vi "Sleep.vi"(8 "error in (no error)":errorcluster, 11 "CIFCorePlugin in":refnum<class "CIFCorePlugin.lvclass">) -> (0 "error out":errorcluster, 2 "Housekeep only":bool, 3 "CIFCorePlugin out":refnum<class "CIFCorePlugin.lvclass">)   [LabVIEW 2021, in "CIFCorePlugin.lvclass"]
uses:
  CIFCorePlugin.lvclass
  CIFCorePlugin.lvclass/CIFCorePlugin.ctl
  CIFUtilities/CIFClocks/Typedef/Errors.ctl
  Accessors/Read Sleep Limits (ns).vi
  Accessors/Timestamps/Write Target Wake TS.vi
  Accessors/Get Time.vi
  Accessors/Timestamps/Read Running TS.vi
  Accessors/Read Running Internal Data.vi
  Accessors/Read Timing Override.vi
  Accessors/Read Common Config.vi
  CIFUtilities/CIFClocks/Core/Get Time.vi
  Common/Utilities/Append Error Location.vi
  CIFUtilities/CIFClocks/Time Conversion/LabVIEW Time to UTC Time.vi
  Common/CIFCoreCommon.lvlib
  CIFUtilities/CIFClocks/CIFClocks.lvlib
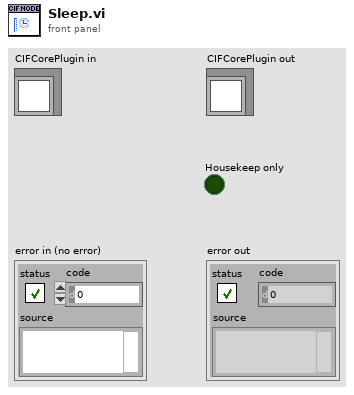
[diagram p1: front panel]
types:
  T1 = typedef "CIFCoreCommon.lvlib/Errors.ctl" = enum16{"Invalid Clock ID", "Long Sleep", "gRPC Server Not Found", "Config Parse", "Timestamp Wrap", "Delayed Execution", "Duplicate Channel", "Missing Channel", "Incorrect Type", "Unregistered Enum"}
  T2 = typedef "CIFCoreCommon.lvlib/Timing Overrides.ctl" = cluster{"Override Timing":bool, "Skip Sleep":bool, "Period (s)":dbl}
  T3 = typedef "CIFCorePlugin.lvclass/Running Internal Data.ctl" = cluster{"Refresh":bool, "Iterations":i64, "Housekeep only":bool, "Configured period (ns)":i64}
  T4 = typedef "CIFCoreCommon.lvlib/Common Plugin Configuration.ctl" = cluster{"Period (s)":dbl, "Offset (us)":i32, "ClockID":u8, "Priority":i32, "Processor":i32}
  T5 = typedef "CIFClocks.lvlib/Future Time Event Limits.ctl" = cluster{"Maximum":u64, "Minimum":u64}
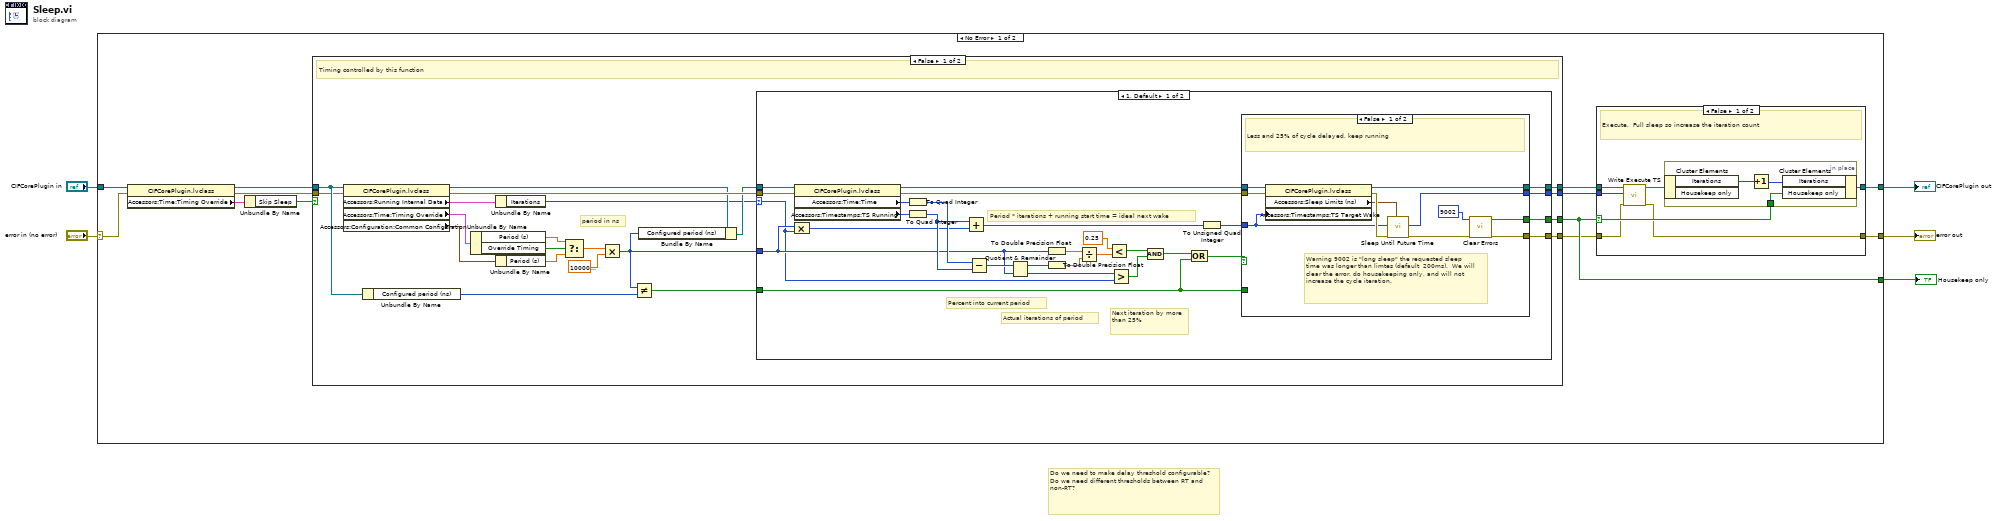
[diagram p0: block diagram]
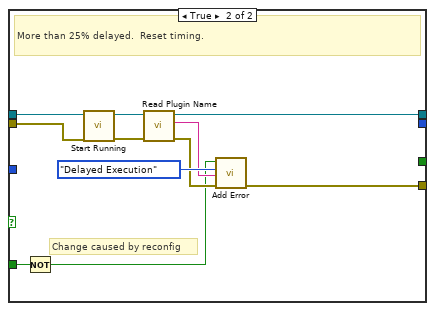
[diagram p2: hidden frame]
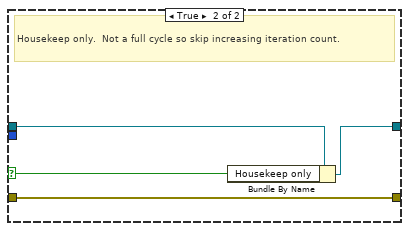
[diagram p5: hidden frame]
diagram:
  # "Do we need to make delay threshold configurable?  Do we need different thresholds between RT and non-RT?"
  n1 = case shown="No Error" "error in (no error)" {
    selector: "error in (no error)" -> [w10 w109]
    tunnel: [w12 w109] -> w4
    tunnel: [w16 w108] -> w2
    tunnel: "CIFCorePlugin in" -> [w11 w108]
    tunnel: [w15 _] -> w1
    frame No Error {
      n2 = property class="CIFCorePlugin.lvclass"(reference=w11, error in=w10) -> (reference out=w9:refnum<class "CIFCorePlugin.lvclass">, error out=w8:errorcluster, "Accessors:Time:Timing Override"=w7:T2)
      n3 = Unbundle By Name(w7) -> ("Skip Sleep"=w6:bool)
      n4 = case shown="False" w6 {
        tunnel: [w38 w93] -> w17
        tunnel: [w24 _] -> w15
        tunnel: [w21 _] -> w14
        tunnel: [w20 w92] -> w13
        tunnel: w9 -> [w19 w93]
        tunnel: w8 -> [w18 w92]
        frame False {
          # "period in ns"
          # "Timing controlled by this function"
          n5 = property class="CIFCorePlugin.lvclass"(reference=w19, error in=w18) -> (reference out=w27:refnum<class "CIFCorePlugin.lvclass">, error out=w37:errorcluster, "Accessors:Running Internal Data"=w23:T3, "Accessors:Time:Timing Override"=w29:T2, "Accessors:Configuration:Common Configuration"=w32:T4)
          n6 = Unbundle By Name(w19) -> ("Configured period (ns)"=w28:i64)
          n7 = Unbundle By Name(w29) -> ("Period (s)"=w31:dbl, "Override Timing"=w33:bool)
          n8 = Unbundle By Name(w32) -> ("Period (s)"=w36:dbl)
          n9 = Unbundle By Name(w23) -> ("Iterations"=w22:i64)
          n10 = Select(t=w31, s=w33, f=w36) -> (s? t:f=w34:dbl)
          n11 = Multiply(x=w34, y=1000000000.0 ("x")) -> (x*y=w25:i64)
          n12 = Not Equal?(x=w25, y=w28) -> (x != y?=w30:bool)
          n13 = Bundle By Name(cluster=w27, "Configured period (ns)"=w25) -> (w26:refnum<class "CIFCorePlugin.lvclass">)
          n14 = case shown="1, Default" w22 {
            selector: w22 -> [w43 _]
            tunnel: [w54 w91] -> w38
            tunnel: w37 -> [w67 w90]
            tunnel: w26 -> [w66 w91]
            tunnel: [w53 w90] -> w20
            tunnel: w25 -> [w45 _]
            tunnel: w30 -> [w47 _]
            tunnel: [w40 _] -> w24
            tunnel: [w39 _] -> w21
            frame 1, Default {
              # "Percent into current period"
              # "Actual iterations of period"
              # "Next iteration by more than 25%"
              # "Period * iterations + running start time = ideal next wake"
              n15 = property class="CIFCorePlugin.lvclass"(reference=w66, error in=w67) -> (reference out=w55:refnum<class "CIFCorePlugin.lvclass">, error out=w52:errorcluster, "Accessors:Time:Time"=w51:u64, "Accessors:Timestamps:TS Running"=w46:u64)
              n16 = Compound Arithmetic op=MULTIPLY(w45, w43) -> (w44:i64)
              n17 = To Quad Integer(1:w51) -> (0:w58:i64)
              n18 = To Quad Integer(1:w46) -> (0:w57:i64)
              n19 = Add(x=w57, y=w44) -> (x+y=w42:i64)
              n20 = Subtract(x=w58, y=w57) -> (x-y=w56:i64)
              n21 = Quotient & Remainder(x=w56, y=w45) -> (x-y*floor(x/y)=w65:i64, floor(x/y)=w50:i64)
              n22 = To Double Precision Float(number=w45) -> (double precision float=w63:dbl)
              n23 = To Double Precision Float(number=w65) -> (double precision float=w64:dbl)
              n24 = Divide(x=w63, y=w64) -> (x/y=w62:dbl)
              n25 = Less?(x=0.25 ("y"), y=w62) -> (x < y?=w60:bool)
              n26 = Greater?(x=w50, y=w43) -> (0:w59:bool)
              n27 = Compound Arithmetic op=AND(w60, w59) -> (w49:bool)
              n28 = Compound Arithmetic op=OR(w49, w47) -> (w48:bool)
              n29 = To Unsigned Quad Integer(1:w42) -> (0:w41:u64)
              n30 = case shown="False" w48 {
                tunnel: w55 -> [w78 w89]
                tunnel: [w71 w84] -> w54
                tunnel: w52 -> [w77 w88]
                tunnel: [w74 w83] -> w53
                tunnel: w47 -> [_ w80]
                tunnel: w41 -> [w69 _]
                tunnel: [w72 _] -> w40
                tunnel: [w70 _] -> w39
                frame False {
                  # "Warning 9002 is \"long sleep\" the requested sleep time was longer than limtes (default  200ms).  We will clear the error, do housekeeping only, and will not increase the cycle iteration."
                  # "Less and 25% of cycle delayed, keep running"
                  n31 = property class="CIFCorePlugin.lvclass"(reference=w78, error in=w77, "Accessors:Timestamps:TS Target Wake"=w69) -> (reference out=w71:refnum<class "CIFCorePlugin.lvclass">, error out=w76:errorcluster, "Accessors:Sleep Limits (ns)"=w68:T5)
                  n32 = call "Sleep Until Future Time.vi"("FTE Limits (ns)"=w68, "error in (no error)"=w76, "Wake Time"=w69) -> ("error out"=w75:errorcluster, "Wake Time (ns)"=w70:u64)  [unwired: 7 in]
                  n33 = call <vilib>:"Clear Errors.vi"("error in (no error)"=w75, "specific error code to clear (0: all)"=9002 ("code")) -> ("error out"=w74:errorcluster, "specific error cleared?"=w72:bool)  [unwired: 4 in]
                }
                frame True {
                  # "Change caused by reconfig"
                  # "More than 25% delayed.  Reset timing."
                  n34 = Not(x=w80) -> (.not. x?=w79:bool)
                  n35 = call "Start Running.vi"("error in (no error)"=w88, "CIFCorePlugin in"=w89) -> ("error out"=w81:errorcluster, "CIFCorePlugin out"=w82:refnum<class "CIFCorePlugin.lvclass">)  [unwired: 8 in]
                  n36 = call "Read Plugin Name.vi"("error in (no error)"=w81, "CIFTemplateNode in"=w82) -> ("error out"=w85:errorcluster, "Plugin Name"=w86:string, "CIFTemplateNode out"=w84:refnum<class "CIFCorePlugin.lvclass">)  [unwired: 7 in]
                  n37 = call "Add Error.vi"("error in (no error)"=w85, "String to Append"=w86, "Error"=Errors."Delayed Execution", "Insert Error"=w79) -> ("error out"=w83:errorcluster)  [unwired: 7 in]
                }
              }
            }
            frame 0 {
              # "First execution when entering running state.  Don't sleep"
            }
          }
        }
        frame True {
          # "Timing Override to skip sleep.  Timing not controlled by this function."
        }
      }
      n38 = case shown="False" w15 {
        selector: w15 -> [w99 w105]
        tunnel: w17 -> [w98 w107]
        tunnel: [w100 w106] -> w16
        tunnel: w14 -> [w96 _]
        tunnel: w13 -> [w95 w104]
        tunnel: [w94 w104] -> w12
        frame False {
          # "Execute.  Full sleep so increase the iteration count"
          n39 = call "Write Execute TS.vi"("error in (no error)"=w95, "Execute"=w96, "CIFCorePlugin in"=w98) -> ("error out"=w94:errorcluster, "CIFCorePlugin out"=w97:refnum<class "CIFCorePlugin.lvclass">)  [unwired: 7 in]
          n40 = in-place {
            in-place-border: w99 -> [w101]
            n41 = in-place-cluster #1(w97) -> ("Iterations"=w102:i64)  [unwired: 1 out]
            n42 = Increment(x=w102) -> (x+1=w103:i64)
            n43 = in-place-cluster #1("Iterations"=w103, "Housekeep only"=w101) -> (w100:refnum<class "CIFCorePlugin.lvclass">)
          }
        }
        frame True {
          # "Housekeep only.  Not a full cycle so skip increasing iteration count."
          n44 = Bundle By Name(cluster=w107, "Housekeep only"=w105) -> (w106:refnum<class "CIFCorePlugin.lvclass">)
        }
      }
    }
    frame Error {
    }
  }
  "error out" <- w4
  "CIFCorePlugin out" <- w2
  "Housekeep only" <- w1
